vi "DestroyPublicEvents.vi"(8 "error in (no error)":errorcluster, 11 "SMO.Example":refnum<class "SMO.Example.lvclass">) -> (0 "error out":errorcluster, 3 "SMO.Example out":refnum<class "SMO.Example.lvclass">)   [LabVIEW 2013, in "SMO.Example.lvclass"]
uses:
  SMO.Example.lvclass
  SMO/SMO.lvclass
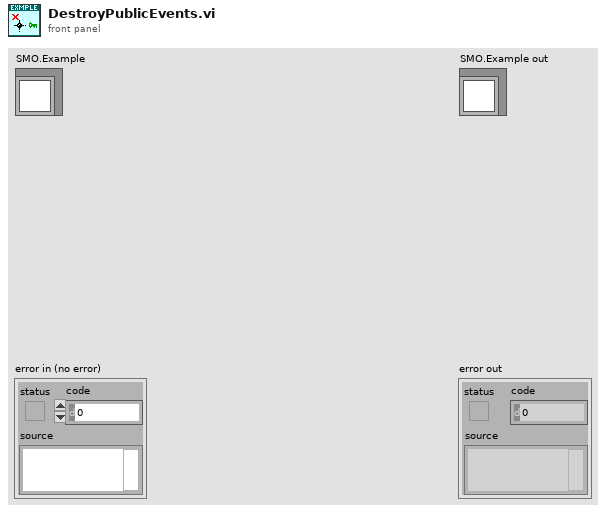
[diagram p1: front panel]
types:
  T1 = typedef "SMO.Example.lvclass/PublicEvents--Cluster.ctl" = cluster{"Data Changed":refnum<user-event>}
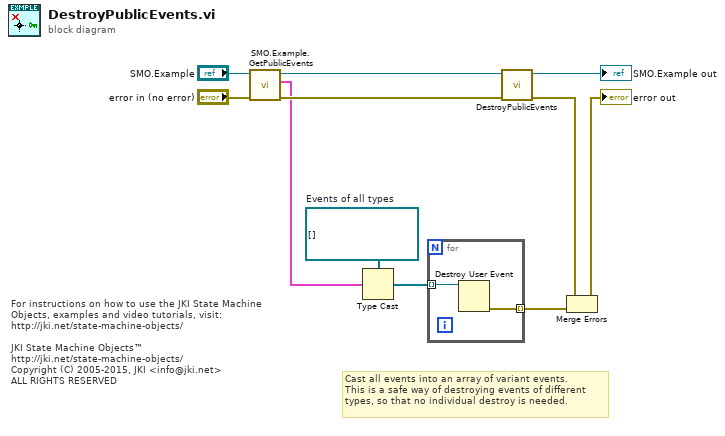
[diagram p0: block diagram]
diagram:
  w6 = refnum<user-event>[] []  # Events of all types
  # "For instructions on how to use the JKI State Machine Objects, examples and video tutorials, visit:\nhttp://jki.net/state-machine-objects/\n\nJKI State Machine Objects™\nhttp://jki.net/state-machine-objects/\nCopyright (C) 2005-2015, JKI <info@jki.net>\nALL RIGHTS RESERVED"
  # "Cast all events into an array of variant events.\nThis is a safe way of destroying events of different\ntypes, so that no individual destroy is needed."
  n1 = call "SMO.Example.GetPublicEvents.vi"("error in (no error)"="error in (no error)", "SMO.Example"="SMO.Example") -> ("error out"=w7:errorcluster, "SMO.Example Public Events"=w3:T1, "SMO.Example out"=w9:refnum<class "SMO.Example.lvclass">)  [unwired: 7 in]
  n2 = Type Cast(type=w6, x=w3) -> (*(type *) &x=w5:refnum<user-event>[])
  n3 = for {
    tunnel: w5 -> [w13] mode=indexing
    tunnel: [w12] -> w4 mode=indexing
    n4 = Destroy User Event(user event=w13) -> (error out=w12:errorcluster)  [unwired: 1 in]
  }
  n5 = call-parent "DestroyPublicEvents.vi"("error in (no error)"=w7, "SMO"=w9) -> ("error out"=w2:errorcluster, "SMO out"=→"SMO.Example out":refnum<class "SMO.Example.lvclass">)  [unwired: 8 in]
  n6 = Merge Errors(w2, w4) -> (→"error out":errorcluster)
